vi "AlliGator Check Missing Python Plugin Doc String.vi"(8 "error in (no error)":errorcluster, 9 "Source":string, 11 "Doc String Found":bool) -> (0 "error out":errorcluster)   [LabVIEW 2021, in "AlliGator Python Plugins.lvlib"]
doc: "Outputs warning with missing doc string message."
uses:
  AlliGator Python Plugins.lvlib
  <vilib>/Utility/error.llb/Error Cluster From Error Code.vi
  <vilib>/ErrorRing/Error Ring.xnode
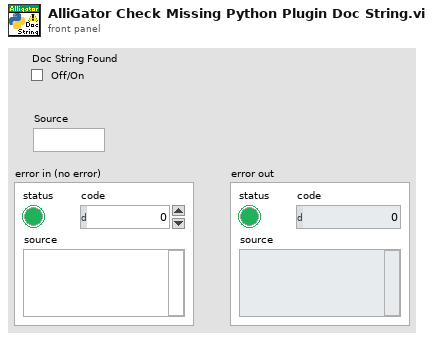
[diagram p1: front panel]
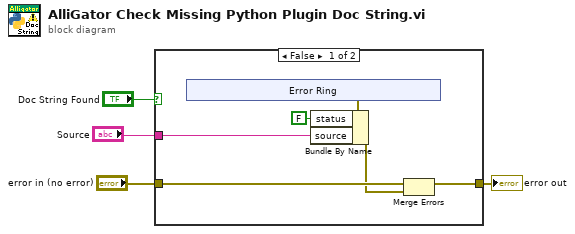
[diagram p0: block diagram]
diagram:
  n1 = case shown="False" "Doc String Found" {
    tunnel: [w10 w15] -> w4
    tunnel: "error in (no error)" -> [w9 w15]
    tunnel: "Source" -> [w5 _]
    frame False {
      n2 = xnode "Error Ring"() -> ("error out"=w6:errorcluster)
      n3 = Bundle By Name(cluster=w6, "status"=FALSE, "source"=w5) -> (w8:errorcluster)
      n4 = Merge Errors(w9, w8) -> (w10:errorcluster)
    }
    frame True {
    }
  }
  "error out" <- w4
